vi "Read Packet.vi"(8 "error in (no error)":errorcluster, 11 "TCPReceiver in":refnum<class "TCPReceiver.lvclass">) -> (0 "error out":errorcluster, 2 "TCPPacket.lvclass":refnum<class "TCPPacket.lvclass">, 3 "TCPReceiver out":refnum<class "TCPReceiver.lvclass">)   [LabVIEW 2019, in "TCPReceiver.lvclass"]
uses:
  TCPReceiver.lvclass
  TCPPacket/TCPPacket.lvclass
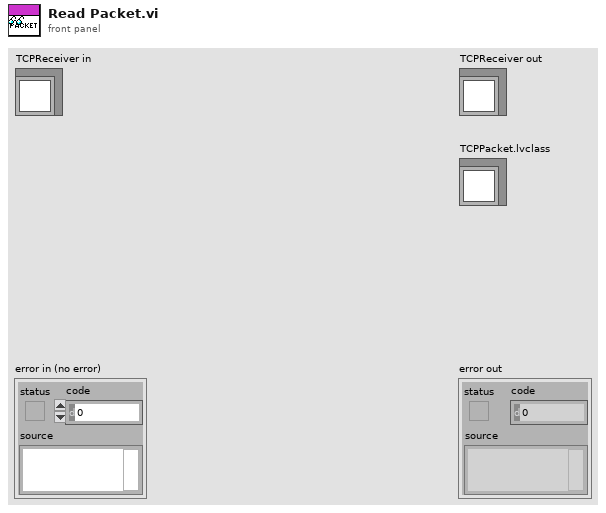
[diagram p1: front panel]
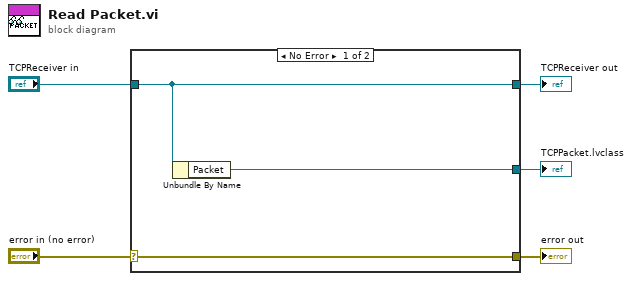
[diagram p0: block diagram]
diagram:
  n1 = case shown="No Error" "error in (no error)" {
    selector: "error in (no error)" -> [w8 w9]
    tunnel: [w8 w9] -> w4
    tunnel: [w7 w10] -> w2
    tunnel: "TCPReceiver in" -> [w7 w10]
    tunnel: [w6 _] -> w1
    frame No Error {
      n2 = Unbundle By Name(w7) -> ("Packet"=w6:refnum<class "TCPPacket.lvclass">)
    }
    frame Error {
    }
  }
  "error out" <- w4
  "TCPReceiver out" <- w2
  "TCPPacket.lvclass" <- w1
